vi "RigolOpticalRabiFlopYB.vi"() -> ()   [LabVIEW 2009]
uses:
  <vilib>/Utility/file.llb/Write To Spreadsheet File (DBL).vi
panel:
  in  "Vpp":dbl
  in  "Stop 1762 Expose (us)":dbl=10.0
  in  "Step Size (us)":dbl=1.0
  out "Current Expose":dbl
  in  "1762 Frequency (MHz)":dbl=9.94 min=0.0 max=30000000.0
  in  "Starting 1762 Expose (us)":dbl=1.0
  in  "Comment":string="Flippin' spins like what"
  in  "B Field":dbl=0.85
  in  "Real Cutoff":dbl=20.0
  out "Shelving Events":dbl=11.0
  out "Dark Counts":dbl=19.0
  out "Bright Counts":dbl=61.0
  in  "Interval":dbl=0.02
  in  "OP Time (us)":dbl=3.0
  in  "Runs per data point":dbl=40.0
  out "Path":path=path "c:/data/1762 Scans/2009-11-09_16-22-05_1762scanWithPumping.txt"
  out "Frequency Scan":cluster{dbl, dbl}[](graph)=[{79100000.0, 0.0}, {79098000.0, 0.01}, {79096000.0, 0.0}, {79094000.0, 0.0}, {79092000.0, 0.0}, {79090000.0, 0.01}, {79088000.0, 0.0}, {79086000.0, 0.0}, {79084000.0, 0.0}, {79082000.0, 0.0}, {79080000.0, 0.0}, {79078000.0, 0.0}, {79076000.0, 0.0}, {79074000.0, 0.02}, {79072000.0, 0.0}, {79070000.0, 0.0}, {79068000.0, 0.0}, {79066000.0, 0.0}, {79064000.0, 0.01}, {79062000.0, 0.0}, {79060000.0, 0.0}, {79058000.0, 0.02}, {79056000.0, 0.01}, {79054000.0, 0.01}, {79052000.0, 0.02}, {79050000.0, 0.01}, {79048000.0, 0.01}, {79046000.0, 0.05}, {79044000.0, 0.01}, {79042000.0, 0.01}, {79040000.0, 0.04}, {79038000.0, 0.02}, {79036000.0, 0.07}, {79034000.0, 0.07}, {79032000.0, 0.04}, {79030000.0, 0.08}, {79028000.0, 0.16}, {79026000.0, 0.22}, {79024000.0, 0.27}, {79022000.0, 0.31}, {79020000.0, 0.37}, {79018000.0, 0.49}, {79016000.0, 0.44}, {79014000.0, 0.36}, {79012000.0, 0.37}, {79010000.0, 0.48}, {79008000.0, 0.23}, {79006000.0, 0.29}, {79004000.0, 0.02}, {79002000.0, 0.02}, {79000000.0, 0.11}]
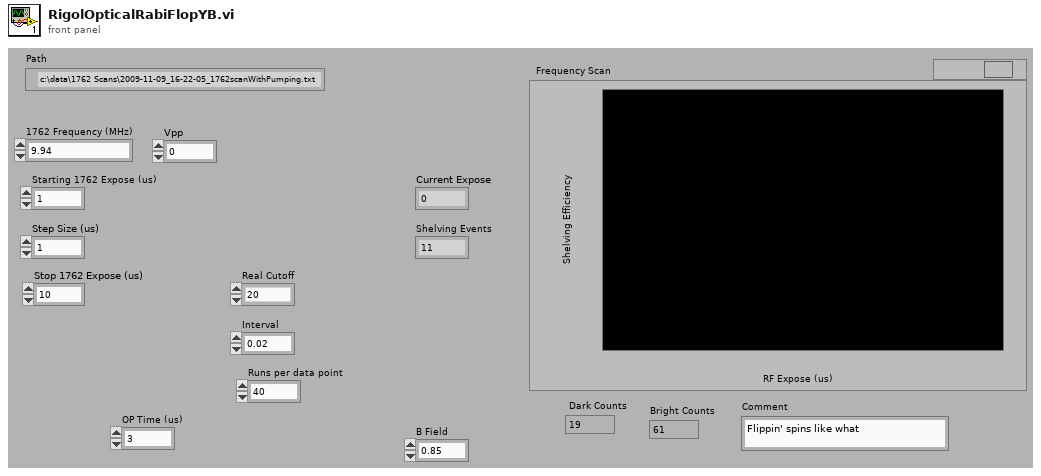
[diagram p1: front panel]
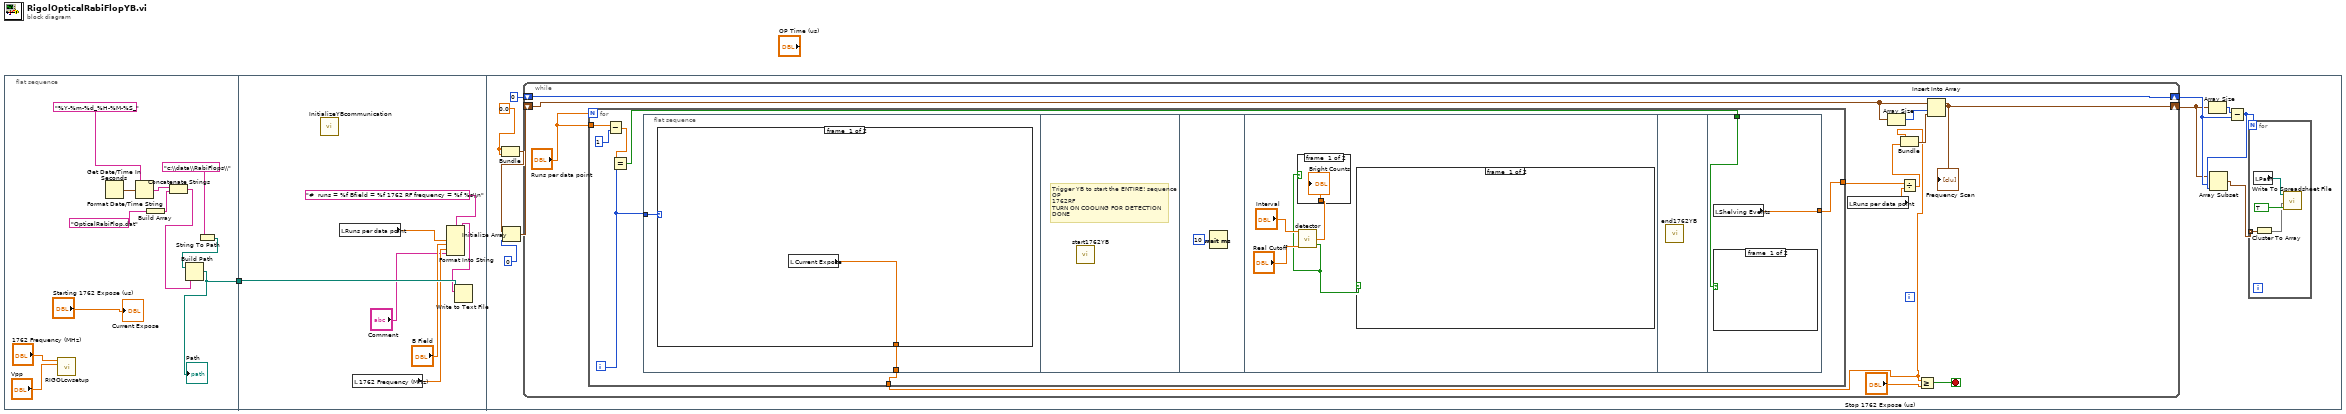
[diagram p0: block diagram]
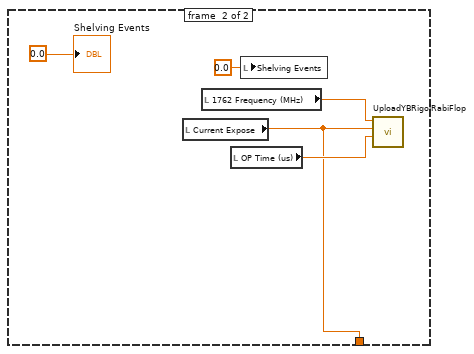
[diagram p2: hidden frame]
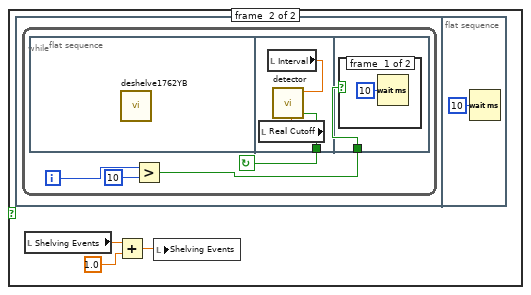
[diagram p3: hidden frame]
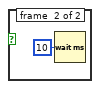
[diagram p4: hidden frame]
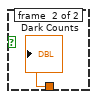
[diagram p5: hidden frame]
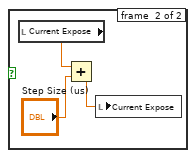
[diagram p6: hidden frame]
diagram:
  n1 = flat-sequence {
    tunnel: [w5] -> w1
    tunnel: w1 -> [w20]
    frame #0 {
      n2 = call "RIGOLcwsetup.vi"("Amplitude (Vpp)"="Vpp", "Frequency (MHz)"="1762 Frequency (MHz)") -> ()  [unwired: 10 in]
      n3 = Get Date/Time In Seconds() -> (seconds since 1Jan1904=w7:timestamp)
      n4 = Format Date/Time String(time format string (%c)="%Y-%m-%d_%H-%M-%S_", seconds (now)=w7) -> (date/time string=w9:string)  [unwired: 1 in]
      n5 = Build Array("OpticalRabiFlop.dat") -> (w12:string[])
      n6 = Concatenate Strings(w9, w12) -> (w11:string)
      n7 = String To Path(string="c:\\data\\RabiFlops\\") -> (path=w13:path)
      n8 = Build Path(base path=w13, name or relative path=w11) -> (appended path=w5:path)
      "Path" <- w5
      "Current Expose" <- "Starting 1762 Expose (us)"
    }
    frame #1 {
      n9 = call "InitializeYBcommunication.vi"() -> ()  [unwired: 12 in]
      n10 = local read "Runs per data point"() -> (w17:dbl)
      n11 = local read "1762 Frequency (MHz)"() -> (w15:dbl)
      n12 = Format Into String(format string="#  runs = %f Bfield = %f 1762 RF frequency = %f %s\\n", w17, "B Field", w15, "Comment") -> (resulting string=w18:string)  [unwired: 2 in, 1 out]
      n13 = Write to Text File(file (use dialog)=w20, text=w18) -> ()  [unwired: 2 in, 3 out]
    }
    frame #2 {
      w29 = 0.0
      n14 = Bundle(w29, w29) -> (w30:cluster{dbl, dbl})  [unwired: 1 in]
      n15 = Initialize Array(w30, 0) -> (w27:cluster{dbl, dbl}[])
      n16 = while {
        shift-right: [w39] -> w22
        shift-left: w27 -> [w41]
        shift-right: [w36] -> w23
        shift-left: 0 -> [w36]
        stop <- w46 stop-if-true
        n17 = for {
          N: "Runs per data point" -> [_]
          tunnel: [w53] -> w45
          tunnel: "Runs per data point" -> [w48]
          tunnel: [w47] -> w35
          i -> [w52]
          n18 = Subtract(x=w48, y=1) -> (x-y=w51:dbl)
          n19 = Equal?(x=w51, y=w52) -> (x = y?=w49:bool)
          n20 = flat-sequence {
            tunnel: w52 -> [w55]
            tunnel: [w54] -> w47
            tunnel: [w84] -> w53
            tunnel: w49 -> [w83]
            frame #0 {
              n21 = case shown="0" w55 {
                tunnel: [w56 w58] -> w54
                frame #0 {
                  n22 = local read "Current Expose"() -> (w56:dbl)
                }
                frame #1 {
                  n23 = local read "Current Expose"() -> (w58:dbl)
                  n24 = local read "1762 Frequency (MHz)"() -> (w61:dbl)
                  n25 = local read "OP Time (us)"() -> (w60:dbl)
                  n26 = local write "Shelving Events"(0.0 ("Shelving Events")) -> ()
                  n27 = call "UploadYBRigolRabiFlop.vi"("OP Time"=w60, "1762 Pulse Time"=w58, "1762 Frequency"=w61) -> ()  [unwired: 9 in]
                  "Shelving Events" <- 0.0 ("Shelving Events")
                }
              }
            }
            frame #1 {
              # "Trigger YB to start the ENTIRE! sequence\nOP\n1762RF\nTURN ON COOLING FOR DETECTION\nDONE"
              n28 = call "start1762YB.vi"() -> ()  [unwired: 11 in, 1 out]
            }
            frame #2 {
              n29 = Wait (ms)(milliseconds to wait=u32 10) -> ()  [unwired: 1 out]
            }
            frame #3 {
              n30 = call "detector.vi"("Cutoff"="Real Cutoff", "Interval"="Interval") -> ("Boolean"=w63:bool, "Counts"=w66:dbl)  [unwired: 3 in]
              n31 = case shown="True" w63 {
                tunnel: w66 -> [w81 w82]
                frame #0 {
                  "Bright Counts" <- w81
                }
                frame #1 {
                  "Dark Counts" <- w82
                }
              }
              n32 = case shown="True" w63 {
                frame #0 {
                }
                frame #1 {
                  n33 = flat-sequence {
                    frame #0 {
                      n34 = while {
                        i -> [w72]
                        stop <- w73 continue-if-true
                        n35 = flat-sequence {
                          tunnel: [w74] -> w73
                          tunnel: w70 -> [w77]
                          frame #0 {
                            n36 = call "deshelve1762YB.vi"() -> ()  [unwired: 11 in, 1 out]
                          }
                          frame #1 {
                            n37 = local read "Real Cutoff"() -> (w75:dbl)
                            n38 = local read "Interval"() -> (w76:dbl)
                            n39 = call "detector.vi"("Cutoff"=w75, "Interval"=w76) -> ("Boolean"=w74:bool)  [unwired: 3 in, 1 out]
                          }
                          frame #2 {
                            n40 = case shown="True" w77 {
                              frame #0 {
                                n41 = Wait (ms)(milliseconds to wait=u32 10) -> ()  [unwired: 1 out]
                              }
                              frame #1 {
                                n42 = Wait (ms)(milliseconds to wait=u32 10) -> ()  [unwired: 1 out]
                              }
                            }
                          }
                        }
                        n43 = Greater?(x=w72, y=10) -> (0:w70:bool)
                      }
                    }
                    frame #1 {
                      n44 = Wait (ms)(milliseconds to wait=u32 10) -> ()  [unwired: 1 out]
                    }
                  }
                  n45 = local read "Shelving Events"() -> (w68:dbl)
                  n46 = Add(x=w68, y=1.0) -> (x+y=w67:dbl)
                  n47 = local write "Shelving Events"(w67) -> ()
                }
              }
            }
            frame #4 {
              n48 = call "end1762YB.vi"() -> ()  [unwired: 1 in]
            }
            frame #5 {
              n49 = local read "Shelving Events"() -> (w84:dbl)
              n50 = case shown="True" w83 {
                frame #0 {
                }
                frame #1 {
                  n51 = local read "Current Expose"() -> (w87:dbl)
                  n52 = Add(x=w87, y="Step Size (us)") -> (x+y=w85:dbl)
                  n53 = local write "Current Expose"(w85) -> ()
                }
              }
            }
          }
        }
        n54 = local read "Runs per data point"() -> (w40:dbl)
        n55 = Array Size(array=w41) -> (size(s)=w44:i32)
        n56 = Divide(x=w45, y=w40) -> (x/y=w42:dbl)
        n57 = Bundle("Current Expose"=w35, w42) -> (w37:cluster{"Current Expose":dbl, dbl})  [unwired: 1 in]
        n58 = Greater Or Equal?(x=w35, y="Stop 1762 Expose (us)") -> (x >= y?=w46:bool)
        n59 = Insert Into Array(array=w41, index=w44, new element=w37) -> (w39:cluster{dbl, dbl}[])
        "Frequency Scan" <- w39
      }
      n60 = Array Size(array=w22) -> (size(s)=w25:i32)
      n61 = Subtract(x=w25, y=w23) -> (x-y=w24:i32)
      n62 = Array Subset(array=w22, index=w23, length=w24) -> (w21:cluster{dbl, dbl}[])
      n63 = for {
        N: w24 -> [_]
        tunnel: w21 -> [w34] mode=indexing
        n64 = local read "Path"() -> (w31:path)
        n65 = Cluster To Array(cluster=w34) -> (array=w32:dbl[])
        n66 = call-poly <vilib>:"Write To Spreadsheet File.vi"("append to file? (new file:F)"=TRUE, "1D data"=w32, "file path (dialog if empty)"=w31) -> ()  [unwired: 5 in, 1 out]
      }
    }
  }
